vi "PhysMon-Read Data Log.vi"(0 "Path":path, 11 "error in (no error)":errorcluster) -> (4 "Notes":string[][](array[string]), 8 "Vital Signs Graph":cluster{"HR Data":cluster{timestamp, dbl}[]}[](array[cluster]), 15 "error out":errorcluster)   [LabVIEW 2020]
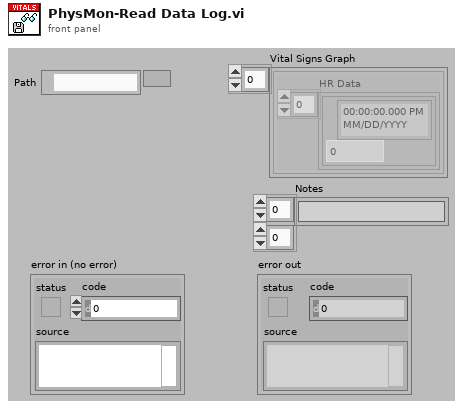
[diagram p1: front panel]
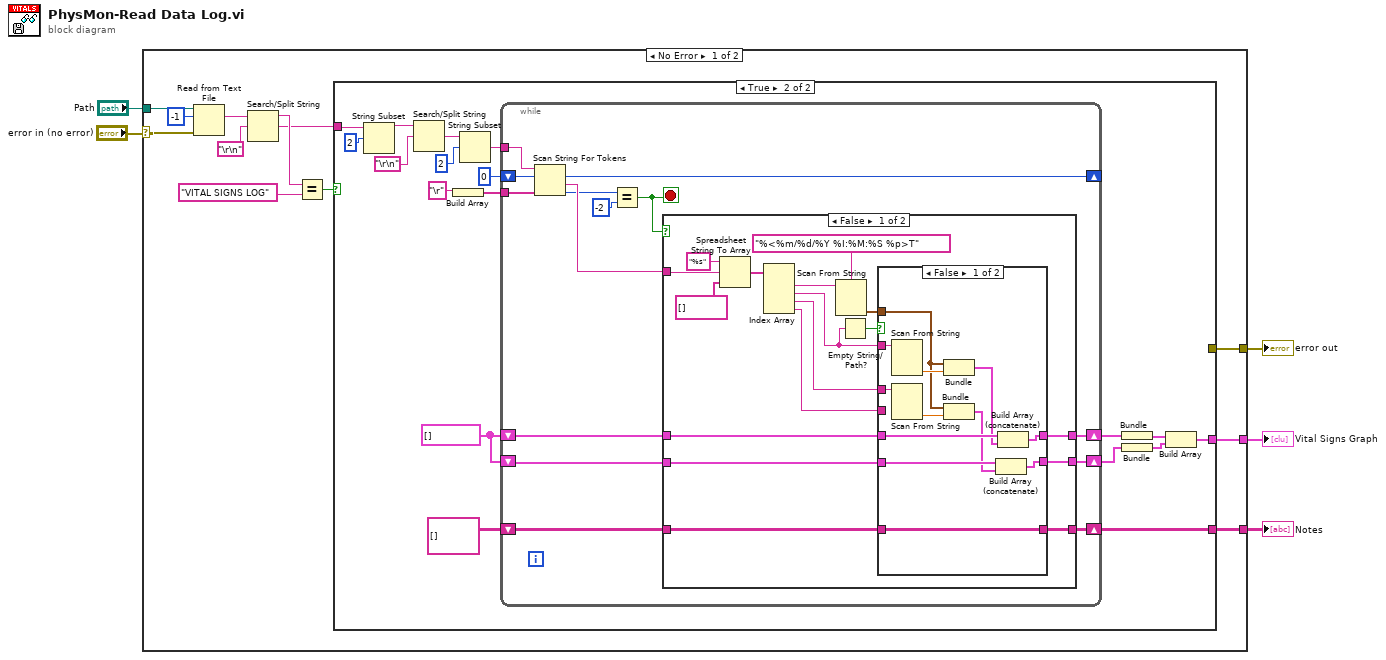
[diagram p0: block diagram]
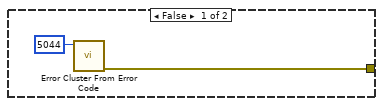
[diagram p2: hidden frame]
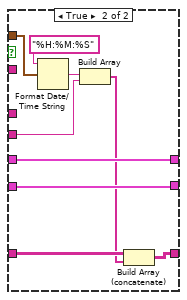
[diagram p3: hidden frame]
diagram:
  n1 = case shown="No Error" "error in (no error)" {
    selector: "error in (no error)" -> [w10 w93]
    tunnel: [w12 w93] -> w4
    tunnel: "Path" -> [w17 _]
    tunnel: [w15 _] -> w2
    tunnel: [w11 _] -> w1
    frame No Error {
      n2 = Read from Text File(file (use dialog)=w17, count=-1, error in=w10) -> (text=w8:string)  [unwired: 1 in, 3 out]
      n3 = Search/Split String(string=w8, search string/char (-)="\r\n") -> (substring before match=w7:string, match + rest of string=w6:string)  [unwired: 1 in, 1 out]
      n4 = Equal?(x=w7, y="VITAL SIGNS LOG") -> (x = y?=w13:bool)
      n5 = case shown="True" w13 {
        tunnel: [_ w35] -> w15
        tunnel: [w18 _] -> w12
        tunnel: [_ w33] -> w11
        tunnel: w6 -> [_ w26]
        frame False {
          n6 = call <vilib>:"Error Cluster From Error Code.vi"("error code (0)"=5044) -> ("error out"=w18:errorcluster)  [unwired: 8 in]
        }
        frame True {
          w21 = cluster{timestamp, dbl}[] []
          n7 = String Subset(string=w26, offset (0)=2) -> (substring=w27:string)  [unwired: 1 in]
          n8 = Search/Split String(string=w27, search string/char (-)="\r\n") -> (match + rest of string=w23:string)  [unwired: 1 in, 2 out]
          n9 = Build Array("\r") -> (w20:string[])
          n10 = String Subset(string=w23, offset (0)=2) -> (substring=w31:string)  [unwired: 1 in]
          n11 = while {
            shift-right: [w50] -> w29
            shift-left: w21 -> [w51]
            shift-right: [w49] -> w28
            shift-left: w21 -> [w48]
            shift-right: [w46] -> w33
            shift-left: string[][] [] -> [w47]
            tunnel: w31 -> [w44]
            shift-right: [w42] -> _
            shift-left: 0 -> [w43]
            tunnel: w20 -> [w38]
            stop <- w39 stop-if-true
            n12 = Scan String For Tokens(6:w38, 8:w43, 9:w44) -> (0:w40:i32, 1:w41:string, 2:w42:i32)  [unwired: 3 in, 1 out]
            n13 = Equal?(x=w40, y=-2 ("x")) -> (x = y?=w39:bool)
            n14 = case shown="False" w39 {
              tunnel: w51 -> [w67 w92]
              tunnel: [w66 w92] -> w50
              tunnel: [w61 w91] -> w49
              tunnel: w48 -> [w60 w91]
              tunnel: w47 -> [w55 w90]
              tunnel: [w54 w90] -> w46
              tunnel: w41 -> [w52 _]
              frame False {
                n15 = Spreadsheet String To Array(format string="%s", spreadsheet string=w52, array type (2D Dbl)=string[] []) -> (array=w63:string[])  [unwired: 1 in]
                n16 = Index Array(array=w63) -> (element #1=w62:string, element #2=w56:string, element #3=w59:string, element #4=w53:string)  [unwired: 4 in]
                n17 = Scan From String(format string="%<%m/%d/%Y %I:%M:%S %p>T", input string=w62) -> (output 1=w58:timestamp)  [unwired: 3 in, 3 out]
                n18 = Empty String/Path?(string/path=w56) -> (empty?=w57:bool)
                n19 = case shown="False" w57 {
                  tunnel: w67 -> [w73 w89]
                  tunnel: [w74 w89] -> w66
                  tunnel: w56 -> [w80 _]
                  tunnel: [w71 w88] -> w61
                  tunnel: w60 -> [w70 w88]
                  tunnel: w59 -> [w78 _]
                  tunnel: w58 -> [w76 w82]
                  tunnel: w55 -> [w75 w84]
                  tunnel: [w75 w83] -> w54
                  tunnel: w53 -> [_ w85]
                  frame False {
                    n20 = Scan From String(input string=w80) -> (output 1=w79:dbl)  [unwired: 4 in, 3 out]
                    n21 = Scan From String(input string=w78) -> (output 1=w77:dbl)  [unwired: 4 in, 3 out]
                    n22 = Bundle(w76, w79) -> (w72:cluster{timestamp, dbl})  [unwired: 1 in]
                    n23 = Bundle(w76, w77) -> (w69:cluster{timestamp, dbl})  [unwired: 1 in]
                    n24 = Build Array (concatenate)(w70, w69) -> (w71:cluster{timestamp, dbl}[])
                    n25 = Build Array (concatenate)(w73, w72) -> (w74:cluster{timestamp, dbl}[])
                  }
                  frame True {
                    n26 = Format Date/Time String(time format string (%c)="%H:%M:%S", seconds (now)=w82) -> (date/time string=w87:string)  [unwired: 1 in]
                    n27 = Build Array(w87, w85) -> (w81:string[])
                    n28 = Build Array (concatenate)(w84, w81) -> (w83:string[][])
                  }
                }
              }
              frame True {
              }
            }
          }
          n29 = Bundle(w29) -> (w37:cluster{cluster{timestamp, dbl}[]})  [unwired: 1 in]
          n30 = Bundle(w28) -> (w36:cluster{cluster{timestamp, dbl}[]})  [unwired: 1 in]
          n31 = Build Array(w37, w36) -> (w35:cluster{cluster{timestamp, dbl}[]}[])
        }
      }
    }
    frame Error {
    }
  }
  "error out" <- w4
  "Vital Signs Graph" <- w2
  "Notes" <- w1
